vi "reset.vi"(8 "error in (no error)":errorcluster, 11 "ScopeNi in":refnum<class "ScopeNi.lvclass">) -> (0 "error out":errorcluster, 3 "ScopeNi out":refnum<class "ScopeNi.lvclass">)   [LabVIEW 2023, in "ScopeNi.lvclass"]
doc: "Reset the instrument to default/factory settings."
uses:
  ScopeNi.lvclass
  ScopeNi.lvclass/ScopeNi.ctl
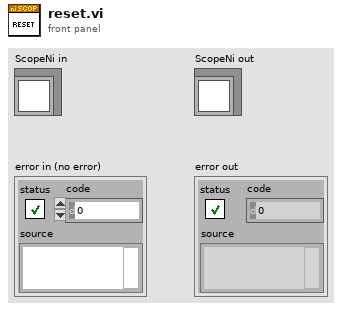
[diagram p1: front panel]
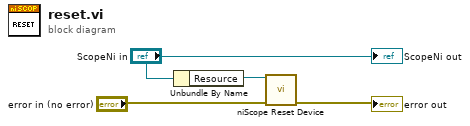
[diagram p0: block diagram]
diagram:
  n1 = Unbundle By Name("ScopeNi in") -> ("Resource"=w3:refnum<k15>)
  n2 = call <instrlib>:"niScope Reset Device.vi"("instrument handle"=w3, "error in"="error in (no error)") -> ("error out"=→"error out":errorcluster)  [unwired: 12 in, 1 out]
  "ScopeNi out" <- "ScopeNi in"
